vi "ProcessResults.vi"(8 "error in (no error)":errorcluster, 11 "Pips in":refnum<class "Pips.lvclass">) -> (0 "error out":errorcluster, 3 "Pips out":refnum<class "Pips.lvclass">)   [LabVIEW 2021, in "Bananas.lvlib" / "Pips.lvclass"]
uses:
  Pips.lvclass
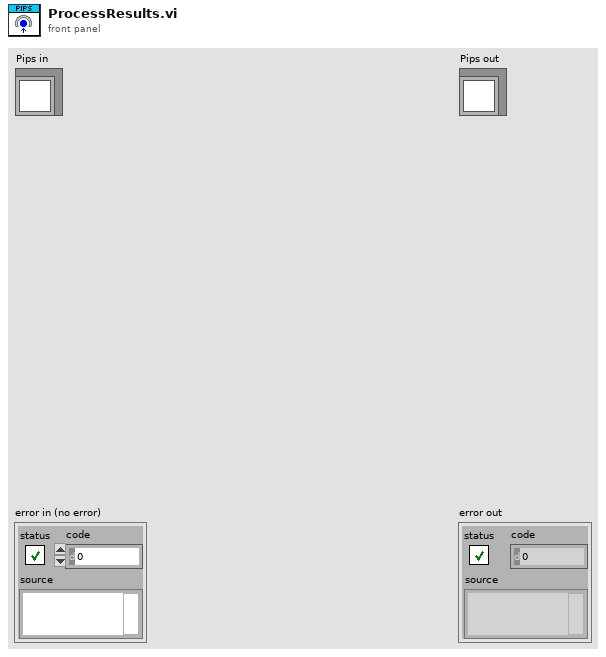
[diagram p1: front panel]
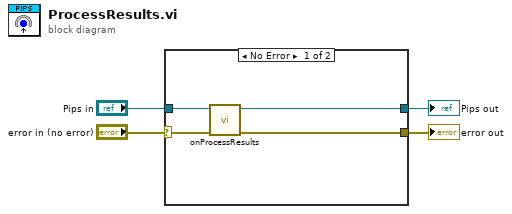
[diagram p0: block diagram]
diagram:
  n1 = case shown="No Error" "error in (no error)" {
    selector: "error in (no error)" -> [w7 w10]
    tunnel: [w6 w10] -> w3
    tunnel: [w5 w9] -> w1
    tunnel: "Pips in" -> [w8 w9]
    frame No Error {
      n2 = call-dynamic "onProcessResults.vi"("error in (no error)"=w7, "Pips in"=w8) -> ("error out"=w6:errorcluster, "Pips out"=w5:refnum<class "Pips.lvclass">)  [unwired: 8 in]
    }
    frame Error {
    }
  }
  "error out" <- w3
  "Pips out" <- w1
